vi "WriteOnePosition.vi"(8 "error in (no error)":errorcluster, 9 "Axis, 1 - 4":i32, 10 "Position, counts":sgl, 11 "UI MotionStatus in":refnum<class "UI MotionStatus.lvclass">) -> (0 "error out":errorcluster, 3 "UI MotionStatus out":refnum<class "UI MotionStatus.lvclass">)   [LabVIEW 2019, in "UI MotionStatus.lvclass"]
uses:
  UI MotionStatus.lvclass
  UI MotionStatus.lvclass/UI MotionStatus.ctl
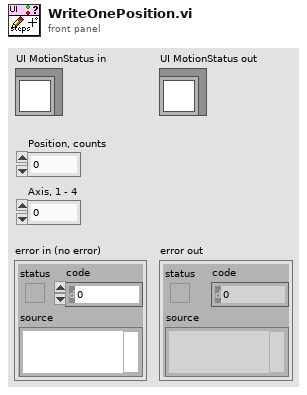
[diagram p1: front panel]
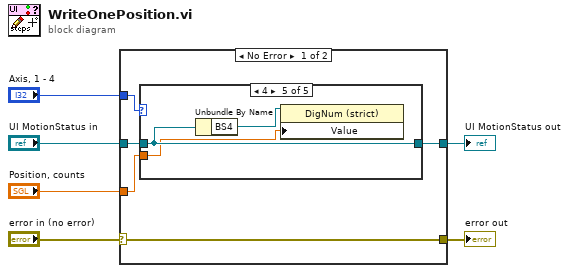
[diagram p0: block diagram]
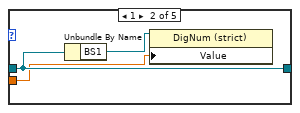
[diagram p3: hidden frame]
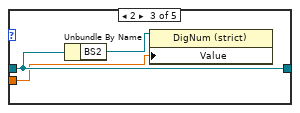
[diagram p4: hidden frame]
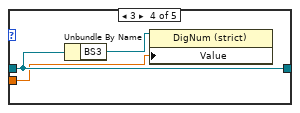
[diagram p5: hidden frame]
diagram:
  n1 = case shown="No Error" "error in (no error)" {
    selector: "error in (no error)" -> [w11 w26]
    tunnel: [w11 w26] -> w5
    tunnel: [w8 w25] -> w3
    tunnel: "UI MotionStatus in" -> [w9 w25]
    tunnel: "Axis, 1 - 4" -> [w10 _]
    tunnel: "Position, counts" -> [w7 _]
    frame No Error {
      n2 = case shown="4" w10 {
        tunnel: [w12 w15 w18 w21 w24] -> w8
        tunnel: w9 -> [w12 w15 w18 w21 w24]
        tunnel: w7 -> [_ w13 w16 w19 w22]
        frame 0, Default {
        }
        frame 1 {
          n3 = Unbundle By Name(w15) -> ("BS1"=w14:refnum<vi>)
          n4 = property class="DigNum (strict)"(reference=w14, "Value"=w13) -> ()  [unwired: 1 in, 2 out]
        }
        frame 2 {
          n5 = Unbundle By Name(w18) -> ("BS2"=w17:refnum<vi>)
          n6 = property class="DigNum (strict)"(reference=w17, "Value"=w16) -> ()  [unwired: 1 in, 2 out]
        }
        frame 3 {
          n7 = Unbundle By Name(w21) -> ("BS3"=w20:refnum<vi>)
          n8 = property class="DigNum (strict)"(reference=w20, "Value"=w19) -> ()  [unwired: 1 in, 2 out]
        }
        frame 4 {
          n9 = Unbundle By Name(w24) -> ("BS4"=w23:refnum<vi>)
          n10 = property class="DigNum (strict)"(reference=w23, "Value"=w22) -> ()  [unwired: 1 in, 2 out]
        }
      }
    }
    frame Error {
    }
  }
  "error out" <- w5
  "UI MotionStatus out" <- w3
